vi "Charge time to Distance.vi"(10 "Charge Time":u64, 11 "Raec Time":u64) -> (3 "Distance":u64)   [LabVIEW 2021, in "Race.lvclass"]
uses:
  Race.lvclass
  Race.lvclass/Race.ctl
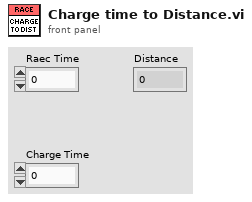
[diagram p1: front panel]
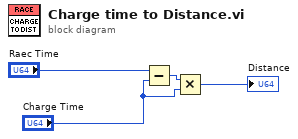
[diagram p0: block diagram]
diagram:
  n1 = Subtract(x="Raec Time", y="Charge Time") -> (x-y=w2:u64)
  n2 = Multiply(x=w2, y="Charge Time") -> (x*y=→"Distance":u64)
